vi "Log Test Result.vi"(8 "error in (no error)":errorcluster, 11 "Sequence Engine in":refnum<class "Sequence Engine.lvclass">) -> (0 "error out":errorcluster, 3 "Sequence Engine out":refnum<class "Sequence Engine.lvclass">)   [LabVIEW 2021]
uses:
  Sequence Engine.lvclass
  Sequence Engine.lvclass/Sequence Engine.ctl
  Report/Classes/Report/Report.lvclass
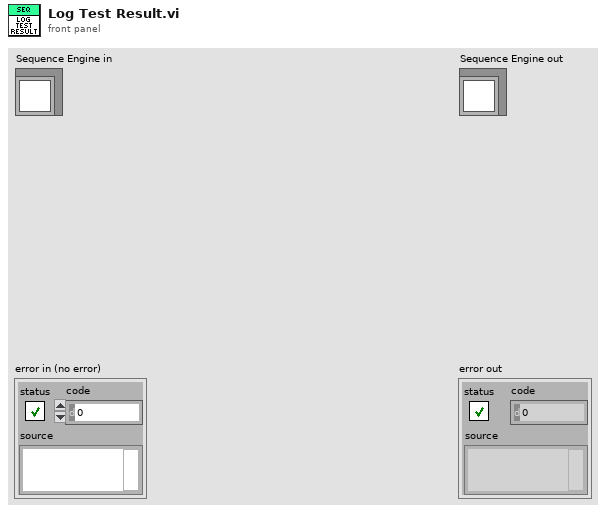
[diagram p1: front panel]
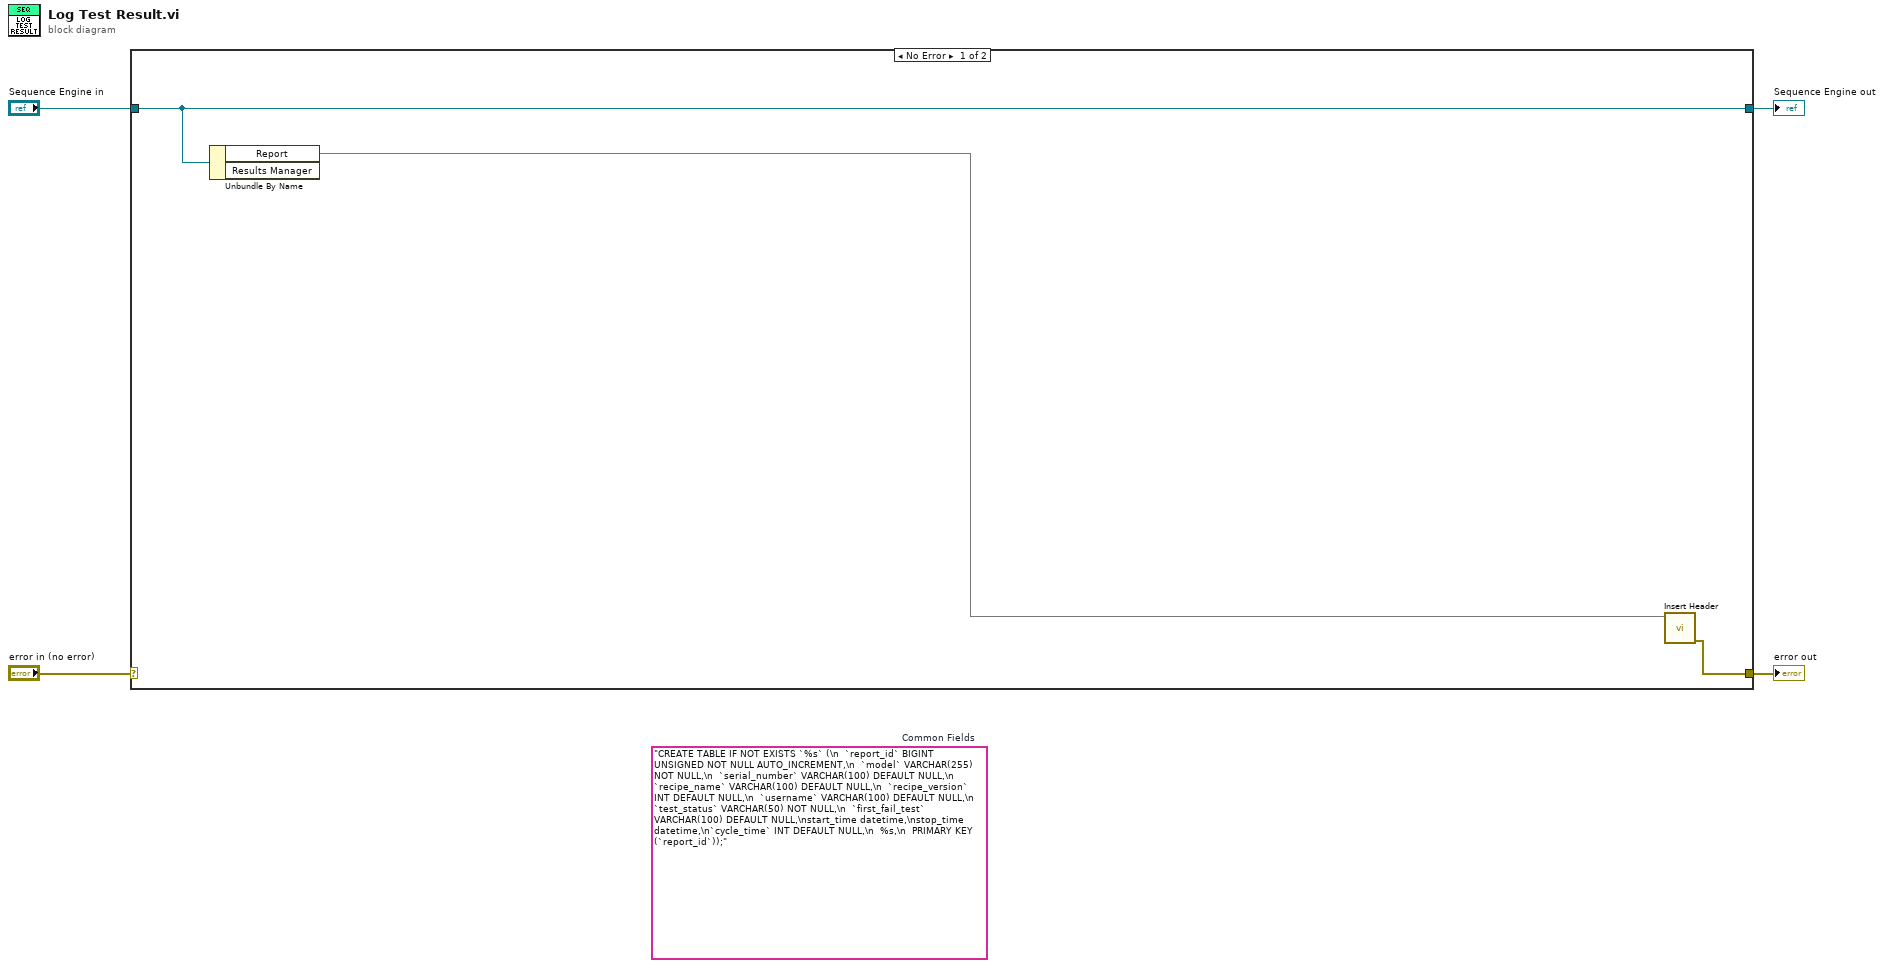
[diagram p0: block diagram]
diagram:
  (unwired) "CREATE TABLE IF NOT EXISTS `%s` (\n  `report_id` BIGINT UNSIGNED NOT NULL AUTO_INCREMENT,\n  `model` VARCHAR(255) NOT NULL,\n  `serial_number` VARCHAR(100) DEFAULT NULL,\n  `recipe_name` VARCHAR(100) DEFAULT NULL,\n  `recipe_version` INT DEFAULT NULL,\n  `username` VARCHAR(100) DEFAULT NULL,\n  `test_status` VARCHAR(50) NOT NULL,\n  `first_fail_test` VARCHAR(100) DEFAULT NULL,\nstart_time datetime,\nstop_time datetime,\n`cycle_time` INT DEFAULT NULL,\n  %s,\n  PRIMARY KEY (`report_id`));"  # Common Fields
  n1 = case shown="No Error" "error in (no error)" {
    selector: "error in (no error)" -> [_ w9]
    tunnel: [w5 w9] -> w3
    tunnel: [w7 w8] -> w1
    tunnel: "Sequence Engine in" -> [w7 w8]
    frame No Error {
      n2 = Unbundle By Name(w7) -> ("Report"=w6)  [unwired: 1 out]
      n3 = call "Insert Header.vi"("Report in"=w6) -> ("error out"=w5:errorcluster)  [unwired: 9 in, 1 out]
    }
    frame Error {
    }
  }
  "error out" <- w3
  "Sequence Engine out" <- w1
